vi "Auto Points.vi"(0 "Char":i16, 7 "Error In":errorcluster) -> (13 "Error Out":errorcluster, 17 "Bottom Goal":dbl, 18 "Top Goal":dbl)   [LabVIEW 2013]
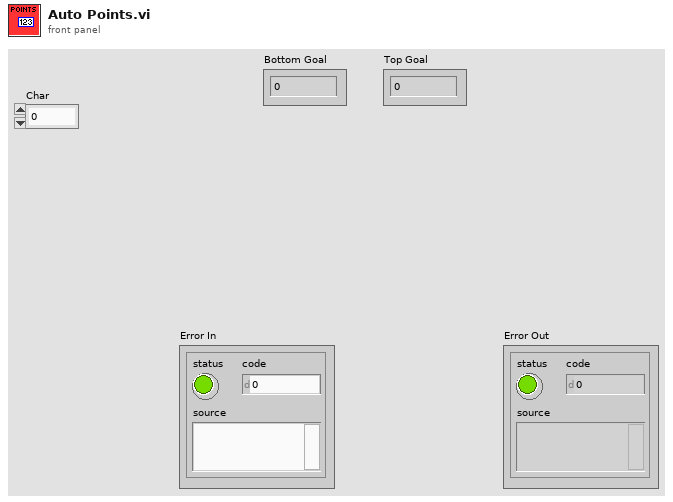
[diagram p1: front panel]
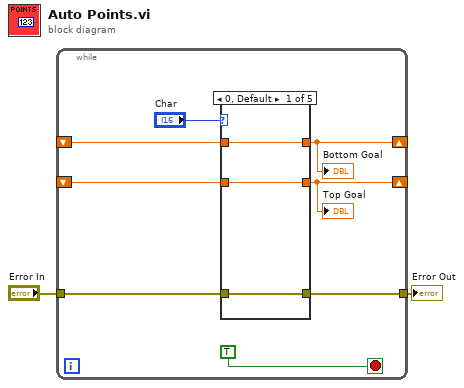
[diagram p0: block diagram]
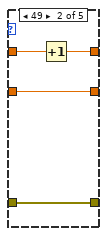
[diagram p2: hidden frame]
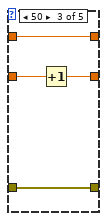
[diagram p3: hidden frame]
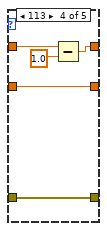
[diagram p4: hidden frame]
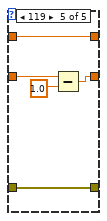
[diagram p5: hidden frame]
diagram:
  n1 = while {
    shift-right: [w8] -> _
    shift-left: _ -> [w10]
    shift-right: [w7] -> _
    shift-left: _ -> [w9]
    tunnel: "Error In" -> [w5]
    tunnel: [w4] -> w1
    stop <- TRUE stop-if-true
    n2 = case shown="0, Default" "Char" {
      tunnel: w10 -> [w13 w16 w21 w25 w31]
      tunnel: w9 -> [w12 w17 w20 w26 w30]
      tunnel: [w12 w17 w19 w26 w28] -> w7
      tunnel: [w13 w15 w21 w23 w31] -> w8
      tunnel: [w11 w14 w18 w22 w27] -> w4
      tunnel: w5 -> [w11 w14 w18 w22 w27]
      frame 0, Default {
      }
      frame 49 {
        n3 = Increment(x=w16) -> (x+1=w15:dbl)
      }
      frame 50 {
        n4 = Increment(x=w20) -> (x+1=w19:dbl)
      }
      frame 113 {
        n5 = Subtract(x=w25, y=1.0) -> (x-y=w23:dbl)
      }
      frame 119 {
        n6 = Subtract(x=w30, y=1.0) -> (x-y=w28:dbl)
      }
    }
    "Bottom Goal" <- w8
    "Top Goal" <- w7
  }
  "Error Out" <- w1
